vi "PFMate-Direct.vi"(2 "Channel":u8=1, 11 "Port":u8=1) -> ()   [LabVIEW 2009]
uses:
  <vilib>/NXT/Subs/LVHSConnector.ctl
panel:
  out "NXT dup":T1={"error"={"status"=FALSE, "code"=0, "source"=""}, "address"="", "NXT #"=-1, "Show Error"=TRUE}
  in  "NXT":T1={"error"={"status"=FALSE, "code"=0, "source"=""}, "address"="", "NXT #"=-1, "Show Error"=TRUE}
  in  "stop":bool
  out "B":bool=TRUE
  out "A":bool=TRUE
  in  "?":bool=TRUE
  in  "?":u8(knob)=5 min=1 max=7 step=1 scale=1.0..7.0
  in  "?":u8(knob)=5 min=1 max=7 step=1 scale=1.0..7.0
  in  "?":u8(ring)
  in  "MB":u8(ring) items=["Run", "Float", "Brake"]
  in  "MA":u8(ring) items=["Run", "Float", "Brake"]
  in  "?":bool=TRUE
  in  "PFMate address":u8=72 caption="PFMate Address" format="%x"
  # "Motor A"
  # "Motor B"
  # "mindsensors.com\nCopyright (c) 2009 by mindsensors.com\nEmail: info (<at>) mindsensors (<dot>) com\n\nThis program is free software. You can redistribute it and/or modify\nit under the terms of the GNU General Public License as published by\nthe Free Software Foundation; version 3 of the License.\nRead the license at: http://www.gnu.org/licenses/gpl.txt"
  # "Mode"
  # "Direction"
  # "Power"
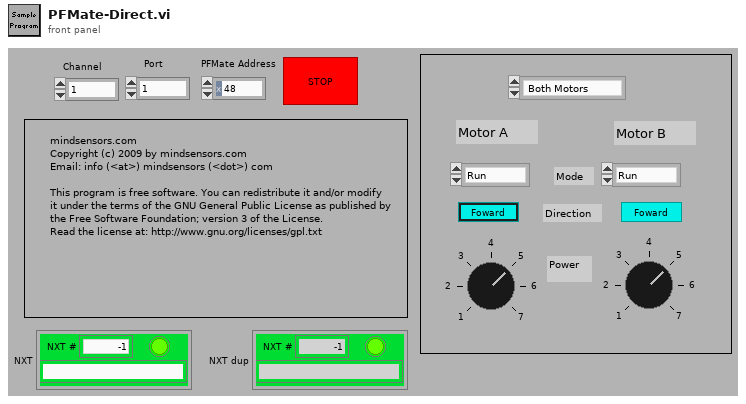
[diagram p1: front panel]
types:
  T1 = typedef "LVHSConnector.ctl" = cluster{"error":errorcluster, "address":string, "NXT #":i32, "Show Error":bool}
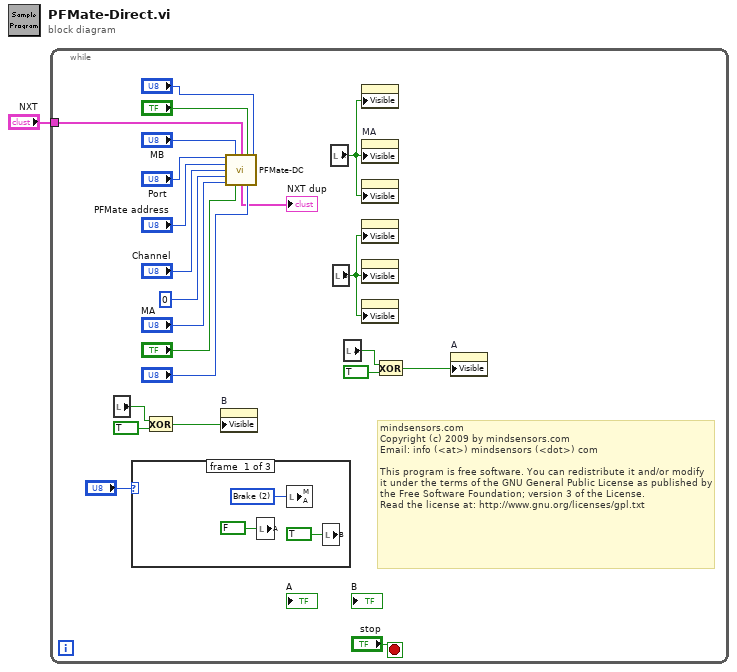
[diagram p0: block diagram]
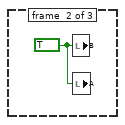
[diagram p2: hidden frame]
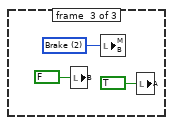
[diagram p3: hidden frame]
diagram:
  n1 = while {
    tunnel: "NXT" -> [w8]
    stop <- "stop" stop-if-true
    # "mindsensors.com\nCopyright (c) 2009 by mindsensors.com\nEmail: info (<at>) mindsensors (<dot>) com\n\nThis program is free software. You can redistribute it and/or modify\nit under the terms of the GNU General Public License as published by\nthe Free Software Foundation; version 3 of the License.\nRead the license at: http://www.gnu.org/licenses/gpl.txt"
    n2 = local read "B"() -> (w11:bool)
    n3 = case shown="2" "?" {
      frame #0 {
        w24 = u8 2 items=["Run", "Float", "Brake"] ("MA")
        n4 = local write "A"(FALSE ("A")) -> ()
        n5 = local write "MA"(w24) -> ()
        n6 = local write "B"(TRUE ("B")) -> ()
      }
      frame #1 {
        w27 = TRUE ("A")
        n7 = local write "B"(w27) -> ()
        n8 = local write "A"(w27) -> ()
      }
      frame #2 {
        w28 = u8 2 items=["Run", "Float", "Brake"] ("MB")
        n9 = local write "B"(FALSE ("B")) -> ()
        n10 = local write "MB"(w28) -> ()
        n11 = local write "A"(TRUE ("A")) -> ()
      }
    }
    n12 = Exclusive Or(1:TRUE ("y"), 2:w11) -> (0:w13:bool)
    n13 = property on="B" class="Boolean"("Visible"=w13) -> ()  [unwired: 2 in, 2 out]
    n14 = call "PFMate-DC.vi"("Connection"="Port", "ModeB"="MB", "NXT"=w8, "DirectionB"="?", "PowerB"="?", "PFMate address"="PFMate address", "Channel"="Channel", "Operate_on"=u8 0, "ModeA"="MA", "DirectionA"="?", "PowerA"="?") -> ("NXT dup"=→"NXT dup":T1)  [unwired: 3 in, 1 out]
    n15 = local read "A"() -> (w6:bool)
    n16 = local read "B"() -> (w5:bool)
    n17 = local read "A"() -> (w2:bool)
    n18 = property class="Boolean (strict)"("Visible"=w6) -> ()  [unwired: 2 in, 2 out]
    n19 = property on="MA" class="Ring (strict)"("Visible"=w6) -> ()  [unwired: 2 in, 2 out]
    n20 = property class="Knob (strict)"("Visible"=w6) -> ()  [unwired: 2 in, 2 out]
    n21 = property class="Boolean (strict)"("Visible"=w5) -> ()  [unwired: 2 in, 2 out]
    n22 = property on="MB" class="Ring (strict)"("Visible"=w5) -> ()  [unwired: 2 in, 2 out]
    n23 = property class="Knob (strict)"("Visible"=w5) -> ()  [unwired: 2 in, 2 out]
    n24 = Exclusive Or(1:TRUE ("y"), 2:w2) -> (0:w4:bool)
    n25 = property on="A" class="Boolean"("Visible"=w4) -> ()  [unwired: 2 in, 2 out]
  }
